vi "Write ActiveDevice.vi"(8 "error in (no error)":errorcluster, 10 "ActiveDevice":refnum<k21>, 11 "SLSC Remote in":refnum<class "SLSC Remote.lvclass">) -> (0 "error out":errorcluster, 3 "SLSC Remote out":refnum<class "SLSC Remote.lvclass">)   [LabVIEW 2016, in "SLSC Interfaces.lvlib" / "SLSC Remote.lvclass"]
uses:
  SLSC Remote.lvclass
  <vilib>/rajsite/i3-json/JSON Generation/Create Value Files/Create Value - String.vi
  <vilib>/rajsite/i3-json/i3-json.lvlib
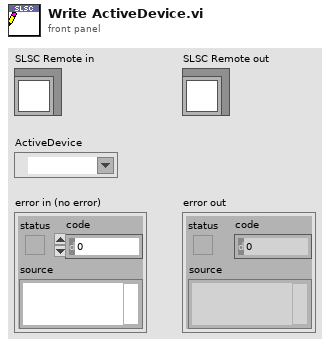
[diagram p1: front panel]
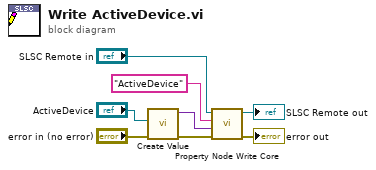
[diagram p0: block diagram]
diagram:
  n1 = call-poly <vilib>:"Create Value.vi"("error in (no error)"="error in (no error)", "String"="ActiveDevice") -> ("error out"=w3:errorcluster, "JSON Tree"=w5:variant)  [unwired: 8 in]
  n2 = call "Property Node Write Core.vi"("error in (no error)"=w3, "value"=w5, "property"="ActiveDevice", "SLSC Remote in"="SLSC Remote in") -> ("error out"=→"error out":errorcluster, "SLSC Remote out"=→"SLSC Remote out":refnum<class "SLSC Remote.lvclass">)  [unwired: 6 in]
